vi "Update-references.vi"(8 "error in (no error)":errorcluster, 9 "Sorted splitter references":refnum<vi>[](array[refnum]), 10 "Sorted pane references":refnum<vi>[](array[refnum]), 11 "Panes in":T1) -> (0 "error out":errorcluster, 3 "Panes out":T1)   [LabVIEW 2013, in "PaneToggle.lvlib" / "Panes.lvclass"]
uses:
  Panes.lvclass
  Object-reference.ctl
  Panes.lvclass/Panes.ctl
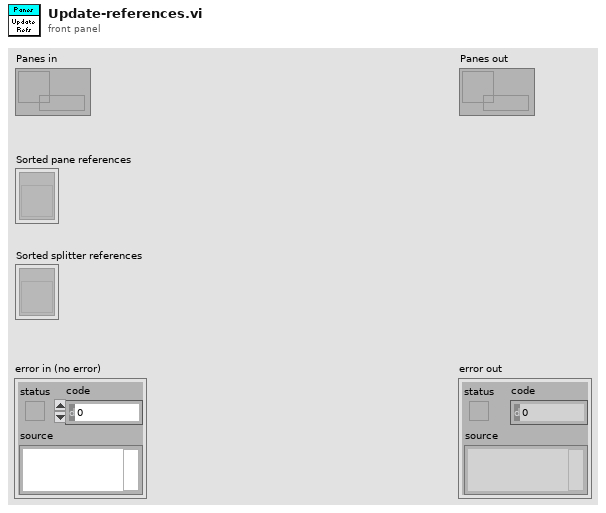
[diagram p1: front panel]
types:
  T1 = typedef "PaneToggle.lvlib/Panes.lvclass/Object-reference.ctl" = refnum<data-value>
  T2 = typedef "PaneToggle.lvlib/Panes.lvclass/Pane-settings.ctl" = cluster{"Pane-name":T3, "Startup visible?":bool, "Currently visible?":bool, "Splitters":T4[], "Pane-reference":refnum<vi>}
  T3 = typedef "PaneToggle.lvlib/Panes.lvclass/Pane-names.ctl" = enum16{"Toolbar", "Help bar", "Toolbar lower border", "Main panel", "Status bar upper border", "General state bar", "Information bar"}
  T4 = typedef "PaneToggle.lvlib/Panes.lvclass/Splitter-settings.ctl" = cluster{"Splitter-name":T5, "Position shown":i32, "Position hidden":i32, "Splitter reference":refnum<vi>}
  T5 = typedef "PaneToggle.lvlib/Panes.lvclass/Splitter-names.ctl" = enum16{"Upper toolbar splitter", "Help bar splitter", "Lower toolbar splitter", "Upper status bar splitter", "Lower status bar splitter", "Left status bar splitter"}
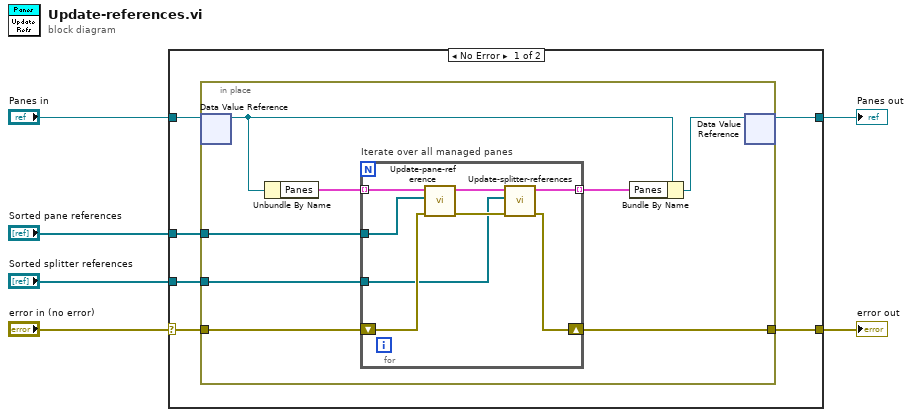
[diagram p0: block diagram]
diagram:
  n1 = case shown="No Error" "error in (no error)" {
    selector: "error in (no error)" -> [w11 w29]
    tunnel: [w10 w29] -> w5
    tunnel: [w7 w30] -> w3
    tunnel: "Panes in" -> [w8 w30]
    tunnel: "Sorted pane references" -> [w12 _]
    tunnel: "Sorted splitter references" -> [w9 _]
    frame No Error {
      n2 = in-place {
        in-place-border: w12 -> [w20]
        in-place-border: w11 -> [w19]
        in-place-border: [w18] -> w10
        in-place-border: w9 -> [w17]
        n3 = in-place-dvr #1(w8) -> (w14:refnum<class "Panes.lvclass">)  [unwired: 1 out]
        n4 = Unbundle By Name(w14) -> ("Panes"=w16:T2[])
        n5 = for "Iterate over all managed panes" {
          tunnel: w16 -> [w27] mode=indexing
          tunnel: w20 -> [w28]
          tunnel: w17 -> [w22]
          tunnel: [w24] -> w15 mode=indexing
          shift-right: [w21] -> w18
          shift-left: w19 -> [w26]
          n6 = call "Update-pane-reference.vi"("error in (no error)"=w26, "Sorted pane references"=w28, "Pane in"=w27) -> ("error out"=w23:errorcluster, "Pane out"=w25:T2)  [unwired: 7 in]
          n7 = call "Update-splitter-references.vi"("error in (no error)"=w23, "Sorted splitter references"=w22, "Pane in"=w25) -> ("error out"=w21:errorcluster, "Pane out"=w24:T2)  [unwired: 7 in]
        }
        n8 = Bundle By Name(cluster=w14, "Panes"=w15) -> (w13:refnum<class "Panes.lvclass">)
        n9 = in-place-dvr #1(w13) -> (w7:T1)  [unwired: 1 out]
      }
    }
    frame Error {
    }
  }
  "error out" <- w5
  "Panes out" <- w3
